vi "ParseDashboardInstruction.vi"(10 "PyramidPosition":string) -> (2 "ArrayInstructions":T1[](array[typedef]))   [LabVIEW 2012]
uses:
  AutoInstruction.ctl
panel:
  in  "AutoInstruction":T1
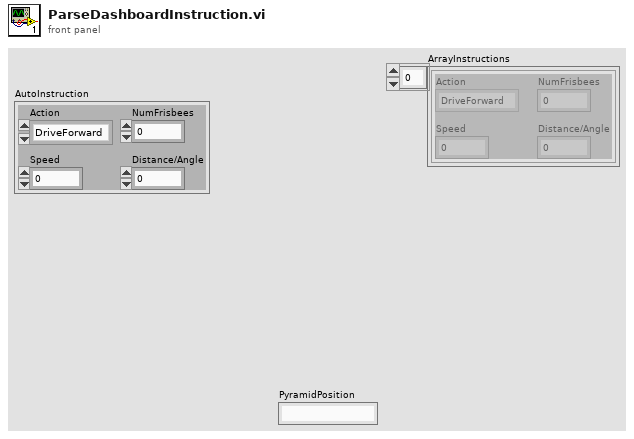
[diagram p1: front panel]
types:
  T1 = typedef "AutoInstruction.ctl" = cluster{"Distance/Angle":dbl, "Speed":dbl, "Action":enum16{"DriveForward", "Turn", "Aim", "Shoot"}, "NumFrisbees":i32}
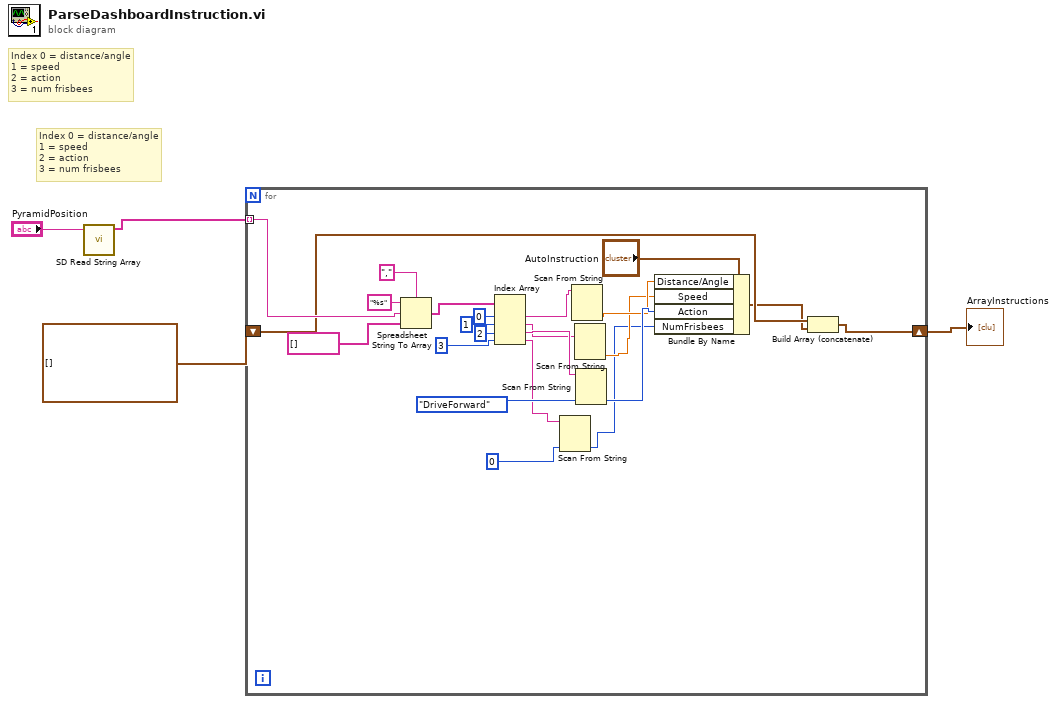
[diagram p0: block diagram]
diagram:
  # "Index 0 = distance/angle\n1 = speed\n2 = action\n3 = num frisbees"
  # "Index 0 = distance/angle\n1 = speed\n2 = action\n3 = num frisbees"
  n1 = call <vilib>:"SD Read String Array.vi"("Name"="PyramidPosition") -> ("String Array"=w1:string[])  [unwired: 9 in, 1 out]
  n2 = for {
    tunnel: w1 -> [w25] mode=indexing
    shift-right: [w13] -> w2
    shift-left: T1[] [] -> [w14]
    n3 = Spreadsheet String To Array(delimiter (Tab)=",", format string="%s", spreadsheet string=w25, array type (2D Dbl)=string[] [] ("Array")) -> (array=w22:string[])
    n4 = Index Array(array=w22, index #1=0 ("index"), index #2=1 ("index"), index #3=2 ("index"), index #4=3 ("index")) -> (element #1=w11:string, element #2=w9:string, element #3=w17:string, element #4=w7:string)
    n5 = Scan From String(input string=w7, default 1=0) -> (output 1=w6:i32)  [unwired: 3 in, 3 out]
    n6 = Scan From String(input string=w11) -> (output 1=w10:dbl)  [unwired: 4 in, 3 out]
    n7 = Scan From String(input string=w9) -> (output 1=w8:dbl)  [unwired: 4 in, 3 out]
    n8 = Scan From String(input string=w17, default 1=enum16{"DriveForward", "Turn", "Aim", "Shoot"}."DriveForward" ("Action")) -> (output 1=w15:enum16{"DriveForward", "Turn", "Aim", "Shoot"})  [unwired: 3 in, 3 out]
    n9 = Bundle By Name(cluster="AutoInstruction", "Distance/Angle"=w10, "Speed"=w8, "Action"=w15, "NumFrisbees"=w6) -> (w12:T1)
    n10 = Build Array (concatenate)(w14, w12) -> (w13:T1[])
  }
  "ArrayInstructions" <- w2
